vi "CIMAQ_Cumulative_Histogram.vi"(0 "Img":T1, 1 "Percentile 1":sgl=10.0, 2 "Percentile 2":sgl=90.0, 3 "error in (no error)":errorcluster, 4 "Number of Classes":i32=256) -> (7 "Cumulative Histogram":dbl[](array[numeric]), 8 "Percentile 1":sgl, 9 "Percentile 2":sgl, 10 "error out":errorcluster)   [LabVIEW 2017]
uses:
  <vilib>/vision/Image Controls.llb/IMAQ Image.ctl
  <vilib>/vision/NI_Vision_Development_Module.lvlib
  <vilib>/Analysis/NI_AALPro.lvlib
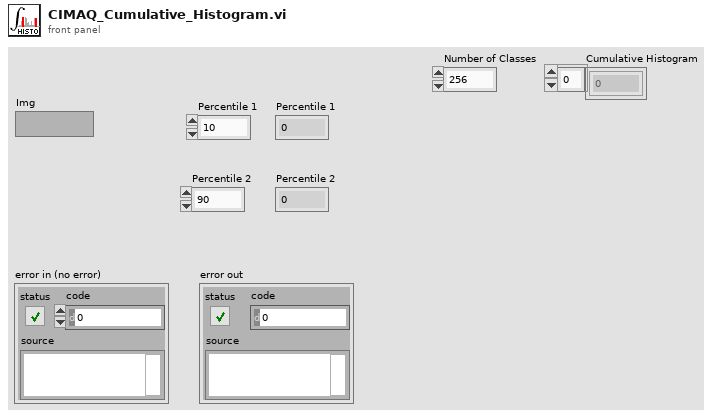
[diagram p1: front panel]
types:
  T1 = typedef "IMAQ Image.ctl" = refnum<image>
  T2 = cluster{"histogram":u32[], "Minimal Value":sgl, "Maximal Value":sgl, "Starting Value":sgl, "Interval Width":sgl, "Mean Value":sgl, "Standard  Variation":sgl, "Area (pixels)":i32}
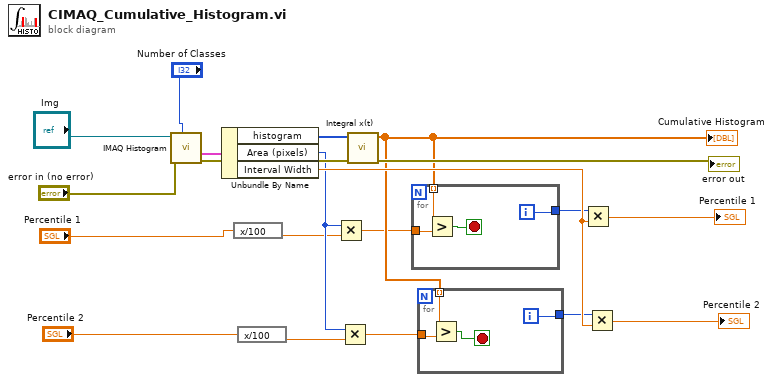
[diagram p0: block diagram]
diagram:
  n1 = call "IMAQ Histogram"("Number of Classes"="Number of Classes", "error in (no error)"="error in (no error)", "Image"="Img") -> ("error out"=→"error out":errorcluster, "Histogram Report"=w2:T2)  [unwired: 7 in]
  n2 = Unbundle By Name(w2) -> ("histogram"=w3:u32[], "Area (pixels)"=w15:i32, "Interval Width"=w19:sgl)
  n3 = expression code="x/100"("Percentile 1") -> (w6:sgl)
  n4 = expression code="x/100"("Percentile 2") -> (w11:sgl)
  n5 = Multiply(x=w15, y=w6) -> (x*y=w7:sgl)
  n6 = Multiply(x=w15, y=w11) -> (x*y=w12:sgl)
  n7 = call <vilib>:"Integral x(t).vi"("X"=w3) -> ("Integral X"=w16:dbl[])  [unwired: 9 in, 1 out]
  "Cumulative Histogram" <- w16
  n8 = for {
    tunnel: w16 -> [w21] mode=indexing
    tunnel: w7 -> [w23]
    tunnel: [w20] -> w8
    i -> [w20]
    stop <- w22 stop-if-true
    n9 = Greater?(x=w21, y=w23) -> (0:w22:bool)
  }
  n10 = for {
    tunnel: w16 -> [w25] mode=indexing
    tunnel: w12 -> [w27]
    tunnel: [w24] -> w13
    i -> [w24]
    stop <- w26 stop-if-true
    n11 = Greater?(x=w25, y=w27) -> (0:w26:bool)
  }
  n12 = Multiply(x=w8, y=w19) -> (x*y=→"Percentile 1":sgl)
  n13 = Multiply(x=w13, y=w19) -> (x*y=→"Percentile 2":sgl)
